vi "GetVelocityArcade.vi"(11 "DriveBase.lvclass":refnum<class "DriveBase.lvclass">) -> (1 "Y Axis":dbl, 2 "X Axis":dbl, 3 "DriveBase.lvclass":refnum<class "DriveBase.lvclass">)   [LabVIEW 2016, in "DriveBase.lvclass"]
uses:
  DriveBase.lvclass
  DriveBase.lvclass/DriveBase.ctl
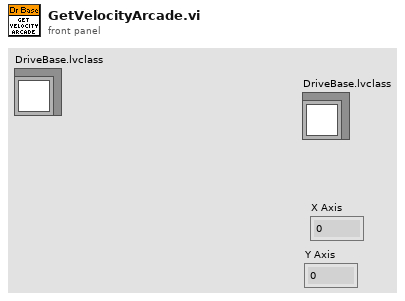
[diagram p1: front panel]
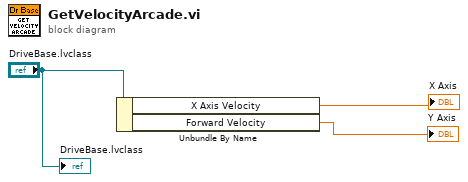
[diagram p0: block diagram]
diagram:
  n1 = Unbundle By Name("DriveBase.lvclass") -> ("X Axis Velocity"=→"X Axis":dbl, "Forward Velocity"=→"Y Axis":dbl)
  "DriveBase.lvclass" <- "DriveBase.lvclass"
